vi "GetConpaneImageData.vi"() -> ()   [LabVIEW 2010]
uses:
  CRef/Core/Master Types.ctl
  <vilib>/Utility/miscctls.llb/LVRectTypeDef.ctl
  CRef/Interface/CRef Boolean.llb/CRef Set Boolean.vi
  CRef/CRef.lvlib
panel:
  out "Array":string[](array[string])
  out "output cluster":T3
  out "Occurance":bool
  out "True Selection":i32
  in  "intSelection":i32
  out "Connector Pane":picture
  out "Terminals":picture
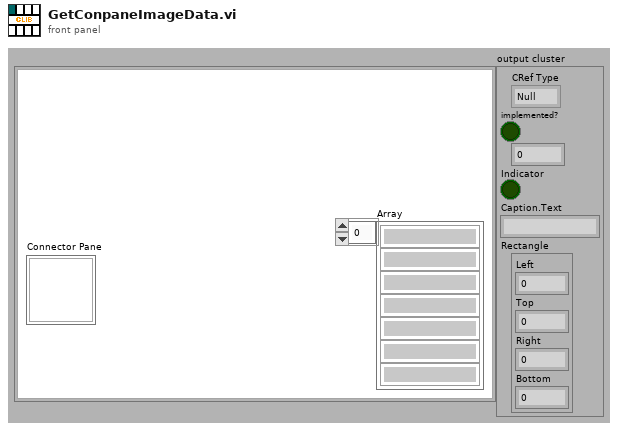
[diagram p1: front panel]
types:
  T1 = typedef "CRef.lvlib/Master Types.ctl" = enum8{"Null", "Boolean", "U8", "I8", "U16", "I16", "U32", "I32", "U64", "I64", "Single", "Double", "Extended", "CSG", "CDB", "CXT", "Boolean(Def)", "U8(Def)", "I8(Def)", "U16(Def)", "I16(Def)", "U32(Def)", "I32(Def)", "Reserved Def", "Reserved Def1", "Single(Def)", "Double(Def)", "Reserved Def2", "Reserved Def3", "Reserved Def4", "Reserved Def5", "Unsigned(Def)", "Signed(Def)", "Real(Def)", "Reserved Def6", "Numeric(Def)", "String"}
  T2 = typedef "LVRectTypeDef.ctl" = cluster{"Left":i16, "Top":i16, "Right":i16, "Bottom":i16}
  T3 = cluster{"CRef Type":T1, "implemented?":bool, i32, "Indicator":bool, "Caption.Text":string, "Rectangle":T2}
  T4 = cluster{"left":i16, "top":i16, "right":i16, "bottom":i16}
  T5 = typedef "imagedata.ctl" = cluster{"image type":i32, "image depth":i32, "image":u8[], "mask":u8[], "colors":u32[], "Rectangle":cluster{"left":i16, "top":i16, "right":i16, "bottom":i16}}
  T6 = cluster{"CRef Type":T1, "implemented?":bool, i32, "Indicator":bool, "Caption.Text":string, "Rectangle":T2}[]
  T7 = typedef "LVPoint32TypeDef.ctl" = cluster{"Horizontal":i32, "Vertical":i32}
  T8 = enum16{"Create", "Get", "Set", "Static", "Release"}
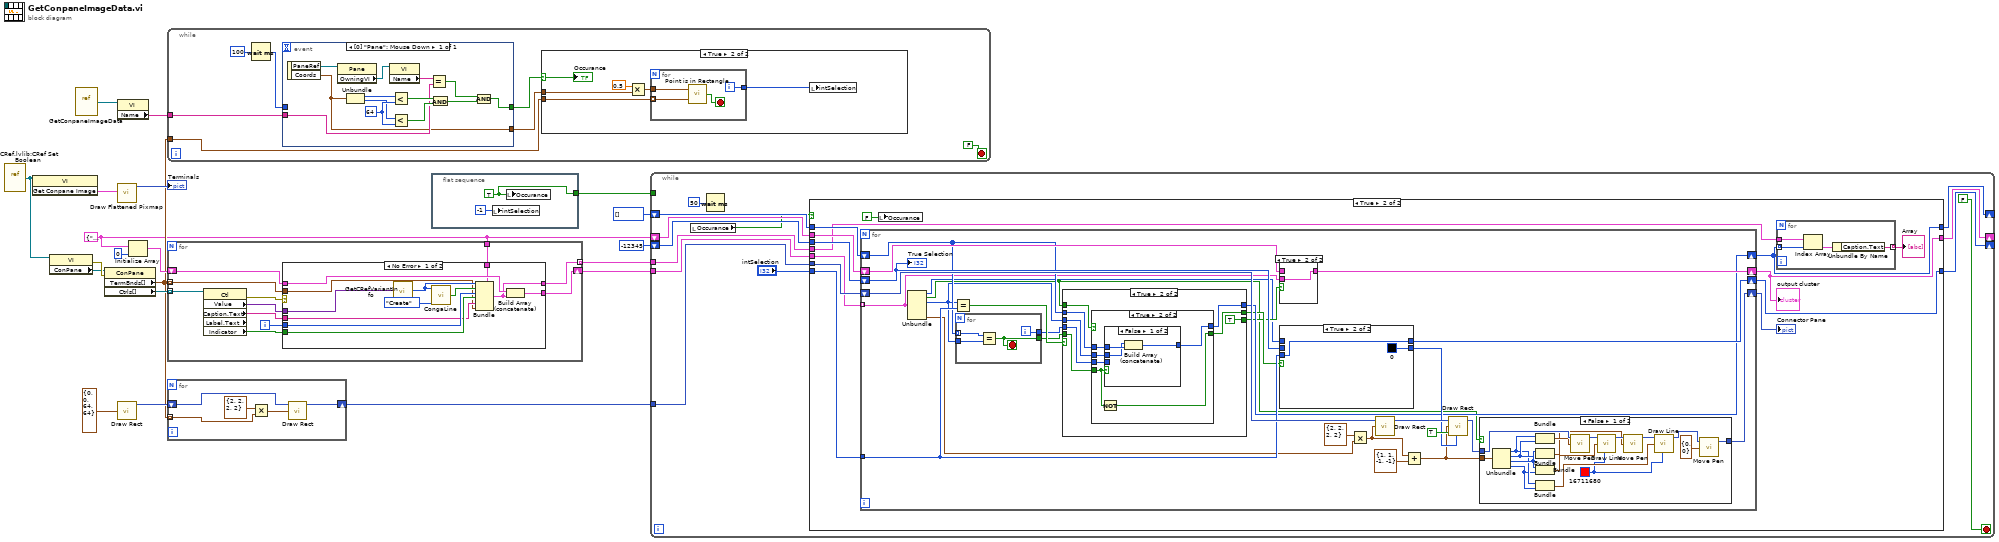
[diagram p0: block diagram]
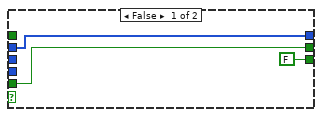
[diagram p6: hidden frame]
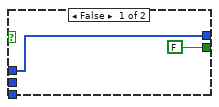
[diagram p7: hidden frame]
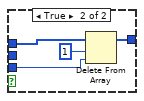
[diagram p8: hidden frame]
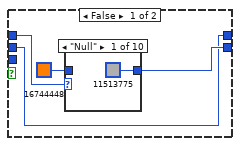
[diagram p9: hidden frame]
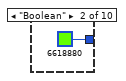
[diagram p10: hidden frame]
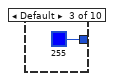
[diagram p11: hidden frame]
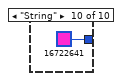
[diagram p18: hidden frame]
diagram:
  w1 = T3 {"CRef Type"=enum."Null", "implemented?"=FALSE, 0, "Indicator"=FALSE, "Caption.Text"="", "Rectangle"={"Left"=0, "Top"=0, "Right"=0, "Bottom"=0}} ("output cluster")
  n1 = vi-ref "CRef.lvlib:CRef Set Boolean.vi"() -> (w16:refnum<vi>)
  n2 = invoke class="VI" method="Get Conpane Image"(reference=w16) -> ("Get Conpane Image"=w18:T5)  [unwired: 2 in, 2 out]
  n3 = property class="VI"(reference=w16) -> (error out=w20:errorcluster, "ConPane"=w19:refnum<vi>)  [unwired: 1 in, 1 out]
  n4 = vi-ref "GetConpaneImageData.vi"() -> (w15:refnum<vi>)
  n5 = property class="ConPane"(reference=w19, error in=w20) -> ("TermBnds[]"=w3:T2[], "Ctrls[]"=w10:refnum<vi>[])  [unwired: 2 out]
  n6 = property class="VI"(reference=w15) -> ("Name"=w14:string)  [unwired: 1 in, 2 out]
  n7 = call <vilib>:"Draw Flattened Pixmap.vi"("image data"=w18) -> ("new picture"=→"Terminals":picture)  [unwired: 8 in]
  n8 = call <vilib>:"Draw Rect.vi"("rect"=T4 {"left"=0, "top"=0, "right"=64, "bottom"=64}) -> ("new picture"=w6:picture)  [unwired: 8 in]
  n9 = Initialize Array(w1, 0 ("dimension size")) -> (w7:T6)
  n10 = while {
    tunnel: w14 -> [w25]
    tunnel: w3 -> [w23]
    stop <- FALSE stop-if-true
    n11 = Wait (ms)(milliseconds to wait=u32 100) -> (millisecond timer value=w21:u32)
    n12 = event shown="[0] \"Pane\": Mouse Down" {
      selector: _ -> [_]
      dyn-events: _ -> [_]
      timeout: _ -> [_]
      tunnel: [w42] -> w24
      tunnel: w25 -> [w39]
      tunnel: [w38] -> w22
      tunnel: w21 -> [_]
      event Mouse Down {
        w47 = 64 ("y")
        n13 = event-data() -> ("PaneRef"=w50:refnum<vi>, "Coords"=w38:T7)  [unwired: 1 in]
        n14 = property class="Pane"(reference=w50) -> ("OwningVI"=w49:refnum<vi>)  [unwired: 1 in, 2 out]
        n15 = Unbundle(w38) -> ("Horizontal"=w41:i32, "Vertical"=w40:i32)
        n16 = property class="VI"(reference=w49) -> ("Name"=w48:string)  [unwired: 1 in, 2 out]
        n17 = Less?(x=w41, y=w47) -> (x < y?=w46:bool)
        n18 = Less?(x=w40, y=w47) -> (x < y?=w45:bool)
        n19 = Equal?(x=w48, y=w39) -> (x = y?=w44:bool)
        n20 = And(x=w46, y=w45) -> (x .and. y?=w43:bool)
        n21 = And(x=w44, y=w43) -> (x .and. y?=w42:bool)
      }
    }
    n22 = case shown="True" w24 {
      selector: w24 -> [_ w28]
      tunnel: w23 -> [_ w33]
      tunnel: w22 -> [_ w32]
      frame False {
      }
      frame True {
        n23 = Multiply(x=0.5, y=w32) -> (x*y=w31:cluster{"Horizontal":dbl, "Vertical":dbl})
        n24 = for {
          tunnel: w33 -> [w37] mode=indexing
          tunnel: w31 -> [w36]
          tunnel: [w35] -> w29
          i -> [w35]
          stop <- w34 stop-if-true
          n25 = call "Point is in Rectangle.vi"("Bounds"=w37, "Point"=w36) -> ("In Bounds?"=w34:bool)
        }
        n26 = local write "intSelection"(w29) -> ()
        "Occurance" <- w28
      }
    }
  }
  n27 = for {
    tunnel: w10 -> [w54] mode=indexing
    shift-right: [w57] -> w9
    shift-left: w7 -> [w55]
    tunnel: w3 -> [w53] mode=indexing
    tunnel: [w52] -> w2 mode=indexing
    tunnel: w1 -> [w51]
    i -> [w60]
    n28 = property class="Ctl" props=["Value", "Caption", "Text", "Label", "Text", "Indicator"](reference=w54) -> (error out=w56:errorcluster, "Value"=w61:variant, "Caption.Text"=w58:string, "Indicator"=w59:bool)  [unwired: 1 in, 2 out]
    n29 = case shown="No Error" w56 {
      tunnel: w61 -> [w72 _]
      tunnel: w60 -> [w69 _]
      tunnel: w59 -> [w68 _]
      tunnel: w58 -> [w67 _]
      tunnel: [w65 w74] -> w57
      tunnel: w55 -> [w66 w74]
      tunnel: w53 -> [w64 _]
      tunnel: [w63 _] -> w52
      tunnel: w51 -> [w62 _]
      frame No Error {
        n30 = call "GetCRefVariantInfo.vi"("variant"=w72) -> ("CRef Type"=w71:T1)  [unwired: 18 in]
        n31 = call "CongaLine.vi"("Type"=w71, "Mode"=T8."Create") -> ("implemented?"=w70:bool)  [unwired: 10 in, 3 out]
        n32 = Bundle(cluster=w62, "CRef Type"=w71, "implemented?"=w70, w69, "Indicator"=w68, "Caption.Text"=w67, "Rectangle"=w64) -> (w63:T3)
        n33 = Build Array (concatenate)(w66, w63) -> (w65:T6)
      }
      frame Error {
      }
    }
  }
  n34 = for {
    shift-right: [w76] -> w4
    shift-left: w6 -> [w79]
    tunnel: w3 -> [w75] mode=indexing
    n35 = Multiply(x=T2 {"Left"=2, "Top"=2, "Right"=2, "Bottom"=2}, y=w75) -> (x*y=w77:T2)
    n36 = call <vilib>:"Draw Rect.vi"("picture"=w79, "rect"=w77) -> ("new picture"=w76:picture)  [unwired: 7 in]
  }
  n37 = flat-sequence {
    tunnel: [w81] -> w11
    frame #0 {
      w81 = TRUE ("Occurance")
      n38 = local write "intSelection"(-1 ("intSelection")) -> ()
      n39 = local write "Occurance"(w81) -> ()
    }
  }
  n40 = while {
    tunnel: w4 -> [w94]
    shift-right: [w92] -> _
    shift-left: -12345 ("Selection") -> [w91]
    shift-right: [w90] -> _
    shift-left: w1 -> [w89]
    shift-right: [w85] -> _
    shift-left: i32[] [] -> [w86]
    tunnel: w11 -> [_]
    tunnel: w9 -> [w83]
    tunnel: w2 -> [w82]
    stop <- FALSE stop-if-true
    n41 = local read "Occurance"() -> (w84:bool)
    n42 = Wait (ms)(milliseconds to wait=u32 50) -> ()  [unwired: 1 out]
    n43 = case shown="True" w84 {
      tunnel: w94 -> [_ w110]
      tunnel: w89 -> [w96 w109]
      tunnel: "intSelection" -> [w97 w108]
      tunnel: [w97 w106] -> w92
      tunnel: w91 -> [_ w105]
      tunnel: [w96 w104] -> w90
      tunnel: w86 -> [w95 w103]
      tunnel: [w95 w101] -> w85
      tunnel: w83 -> [_ w100]
      tunnel: w82 -> [_ w99]
      frame False {
      }
      frame True {
        n44 = for {
          shift-right: [w117] -> w107
          shift-left: w110 -> [w141]
          tunnel: w100 -> [w119] mode=indexing
          shift-right: [w140] -> w104
          shift-left: w109 -> [w139]
          tunnel: w108 -> [w131]
          shift-right: [w130] -> w106
          shift-left: w105 -> [w129]
          shift-right: [w127] -> w101
          shift-left: w103 -> [w128]
          n45 = Unbundle(w119) -> ("CRef Type"=w121:T1, "implemented?"=w116:bool, w120:i32, "Rectangle"=w118:T2)  [unwired: 2 out]
          n46 = Equal?(x=w120, y=w131) -> (x = y?=w126:bool)
          n47 = for {
            tunnel: w128 -> [w191] mode=indexing
            tunnel: [w188] -> w125
            tunnel: [w190] -> w124
            tunnel: w120 -> [w189]
            i -> [w188]
            stop <- w190 stop-if-true
            n48 = Equal?(x=w191, y=w189) -> (x = y?=w190:bool)
          }
          n49 = case shown="True" w126 {
            tunnel: w125 -> [_ w172]
            tunnel: w128 -> [w164 w171]
            tunnel: [w164 w170] -> w127
            tunnel: w124 -> [w162 w169]
            tunnel: [w162 w168] -> w123
            tunnel: w120 -> [_ w167]
            tunnel: w116 -> [_ w166]
            tunnel: [FALSE TRUE] -> w122
            frame False {
            }
            frame True {
              n50 = case shown="True" w166 {
                tunnel: w172 -> [_ w180]
                tunnel: w171 -> [w174 w179]
                tunnel: [w174 w178] -> w170
                tunnel: w169 -> [_ w177]
                tunnel: [FALSE w175] -> w168
                tunnel: w167 -> [_ w176]
                frame False {
                }
                frame True {
                  n51 = Not(x=w177) -> (.not. x?=w175:bool)
                  n52 = case shown="False" w177 {
                    tunnel: w180 -> [_ w187]
                    tunnel: w179 -> [w183 w186]
                    tunnel: [w182 w185] -> w178
                    tunnel: w176 -> [w181 _]
                    frame False {
                      n53 = Build Array (concatenate)(w181, w183) -> (w182:i32[])
                    }
                    frame True {
                      n54 = Delete From Array(array=w186, length=1, index=w187) -> (array with subset deleted=w185:i32[])  [unwired: 1 out]
                    }
                  }
                }
              }
            }
          }
          n55 = case shown="True" w122 {
            tunnel: w139 -> [w160 _]
            tunnel: [w160 w161] -> w140
            tunnel: w119 -> [_ w161]
            frame False {
            }
            frame True {
            }
          }
          n56 = case shown="True" w123 {
            tunnel: [w195 u32 0 ("color(black)")] -> w132
            tunnel: w121 -> [w194 _]
            tunnel: w129 -> [w192 _]
            tunnel: [w192 w206] -> w130
            tunnel: w131 -> [_ w206]
            frame False {
              n57 = case shown="\"Null\"" w194 {
                tunnel: [u32 11513775 ("color(black)") u32 6618880 ("color(black)") u32 255 ("color(black)") w199 w200 w201 w202 w203 w204 u32 16722641 ("color(black)")] -> w195
                tunnel: u32 16744448 ("color(black)") -> [_ _ _ w199 w200 w201 w202 w203 w204 _]
                frame "Null" {
                }
                frame "Boolean" {
                }
                frame Default {
                }
                frame "Single" {
                }
                frame "Double" {
                }
                frame "Extended" {
                }
                frame "CSG" {
                }
                frame "CDB" {
                }
                frame "CXT" {
                }
                frame "String" {
                }
              }
            }
            frame True {
            }
          }
          n58 = Multiply(x=T2 {"Left"=2, "Top"=2, "Right"=2, "Bottom"=2}, y=w118) -> (x*y=w135:T2)
          n59 = call <vilib>:"Draw Rect.vi"("picture"=w141, "rect"=w135) -> ("new picture"=w137:picture)  [unwired: 7 in]
          n60 = Add(x=w135, y=T2 {"Left"=1, "Top"=1, "Right"=-1, "Bottom"=-1}) -> (x+y=w115:T2)
          n61 = call <vilib>:"Draw Rect.vi"("picture"=w137, "rect"=w115, "fill?(F)"=TRUE, "color(black)"=w132) -> ("new picture"=w136:picture)  [unwired: 5 in]
          n62 = case shown="False" w116 {
            tunnel: w136 -> [w156 w159]
            tunnel: [w145 w159] -> w117
            tunnel: w115 -> [w155 _]
            frame False {
              w143 = u32 16711680 ("color(black)")
              n63 = Unbundle(w155) -> ("Left"=w152:i16, "Top"=w153:i16, "Right"=w154:i16, "Bottom"=w151:i16)
              n64 = Bundle("Left"=w152, "Top"=w153) -> (w150:cluster{"Left":i16, "Top":i16})  [unwired: 1 in]
              n65 = Bundle("Right"=w154, "Top"=w153) -> (w148:cluster{"Right":i16, "Top":i16})  [unwired: 1 in]
              n66 = Bundle("Right"=w154, "Bottom"=w151) -> (w149:cluster{"Right":i16, "Bottom":i16})  [unwired: 1 in]
              n67 = Bundle("Left"=w152, "Bottom"=w151) -> (w147:cluster{"Left":i16, "Bottom":i16})  [unwired: 1 in]
              n68 = call <vilib>:"Move Pen.vi"("new position"=w150, "picture"=w156) -> ("new picture"=w142:picture)  [unwired: 3 in]
              n69 = call <vilib>:"Draw Line.vi"("picture"=w142, "end point"=w149, "color(black)"=w143) -> ("new picture"=w158:picture)  [unwired: 6 in]
              n70 = call <vilib>:"Move Pen.vi"("new position"=w148, "picture"=w158) -> ("new picture"=w157:picture)  [unwired: 3 in]
              n71 = call <vilib>:"Draw Line.vi"("picture"=w157, "end point"=w147, "color(black)"=w143) -> ("new picture"=w146:picture)  [unwired: 6 in]
              n72 = call <vilib>:"Move Pen.vi"("new position"=cluster{"x":i16, "y":i16} {"x"=0, "y"=0}, "picture"=w146) -> ("new picture"=w145:picture)  [unwired: 3 in]
            }
            frame True {
            }
          }
          "True Selection" <- w129
        }
        "Connector Pane" <- w107
        "output cluster" <- w104
        n73 = local write "Occurance"(FALSE ("Occurance")) -> ()
        n74 = for {
          tunnel: w101 -> [w114] mode=indexing
          tunnel: w99 -> [w113]
          tunnel: [w111] -> w98 mode=indexing
          n75 = Index Array(array=w113, index=w114) -> (element=w112:T3)
          n76 = Unbundle By Name(w112) -> ("Caption.Text"=w111:string)
        }
        "Array" <- w98
      }
    }
  }
